vi "Send Draw Assert Data.vi"(7 "Message Priority (Normal)":T2=enum."Normal", 8 "error in (no error)":errorcluster, 10 "Assert Array":T1[](array[typedef]), 11 "Message Enqueuer":refnum<class "Message Enqueuer.lvclass">) -> (0 "error out":errorcluster, 3 "Message Enqueuer out":refnum<class "Message Enqueuer.lvclass">)   [LabVIEW 2016, in "UserInterface.lvlib" / "Draw Assert Data Msg.lvclass"]
doc: "This VI sends the message to an actor."
uses:
  Draw Assert Data Msg.lvclass
  <vilib>/ActorFramework/Message Enqueuer/Message Enqueuer.lvclass
  <vilib>/ActorFramework/Message Enqueuer/Message Priority.ctl
  AssertEngine/Log Assert/Assert Data.ctl
  C:/Program Files/National Instruments/LabVIEW 2016/vi.lib/ActorFramework/Message/Message.lvclass
  Draw Assert Data Msg.lvclass/Draw Assert Data Msg.ctl
  <vilib>/ActorFramework/Message Enqueuer/Message Enqueuer.lvclass/Message Enqueuer.ctl
  <vilib>/ActorFramework/Message Priority Queue/Priority Enqueue.vi
  AssertEngine/AssertEngine.lvlib
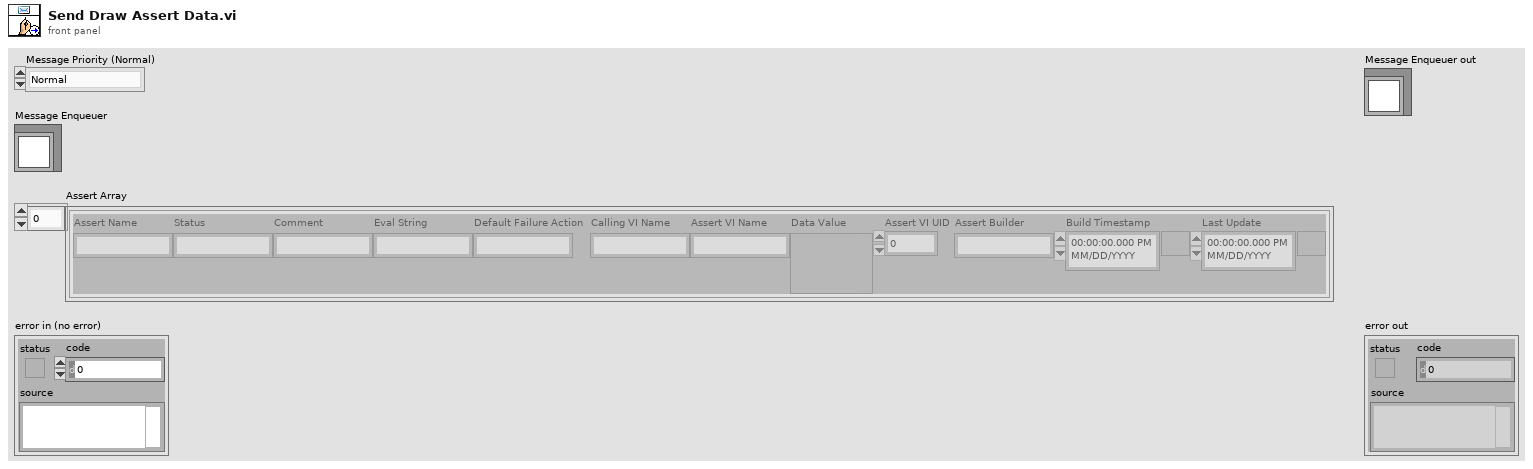
[diagram p1: front panel]
types:
  T1 = typedef "AssertEngine.lvlib/Assert Data.ctl" = cluster{"Assert Name":string, "Status":string, "Comment":string, "Eval String":string, "Default Failure Action":string, "Calling VI Name":string, "Assert VI Name":string, "Data Value":variant, "Assert VI UID":i32, "Assert Builder":string, "Build Timestamp":timestamp, "Last Update":timestamp}
  T2 = typedef "Actor Framework.lvlib/Message Enqueuer.lvclass/Message Priority.ctl" = enum16{"Low", "Normal", "High"}
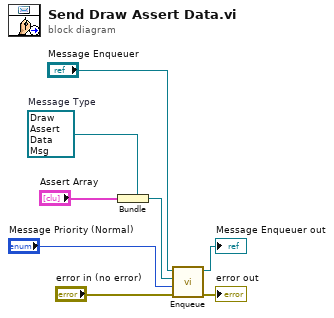
[diagram p0: block diagram]
diagram:
  w2 = refnum<class "Draw Assert Data Msg.lvclass"> refnum  # Message Type
  n1 = Bundle(cluster=w2, "Assert Array") -> (w3:refnum<class "Draw Assert Data Msg.lvclass">)
  n2 = call <vilib>:"Enqueue.vi"("error in (no error)"="error in (no error)", "Message Priority (Normal)"="Message Priority (Normal)", "Message"=w3, "Message Enqueuer in"="Message Enqueuer") -> ("error out"=→"error out":errorcluster, "Message Enqueuer out"=→"Message Enqueuer out":refnum<class "Message Enqueuer.lvclass">)  [unwired: 6 in]
